vi "read data.vi"() -> ()   [LabVIEW 2017]
panel:
  out "size(s)":i32
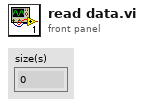
[diagram p1: front panel]
types:
  T1 = cluster{"RTDs":dbl[], "Thermocouples":dbl[], "Pressure Transducers":dbl[], "Mass Flow Meters":dbl[], "Barometer":dbl[], "Accelerometer":dbl[], "Current ":dbl[]}
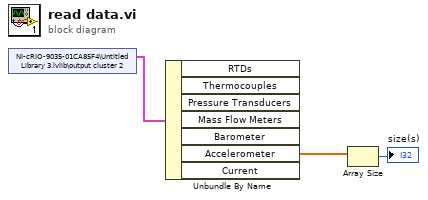
[diagram p0: block diagram]
diagram:
  n1 = shared-variable "NI-cRIO-9035-01CA85F4\\Untitled Library 3.lvlib\\output cluster 2"() -> (w3:T1)  [unwired: 1 in, 1 out]
  n2 = Unbundle By Name(w3) -> ("Accelerometer"=w2:dbl[])  [unwired: 6 out]
  n3 = Array Size(array=w2) -> (size(s)=→"size(s)":i32)
